vi "Cylinder Chart View.vi"(10 "User Events in":refnum<class "User Events.lvclass">) -> ()   [LabVIEW 2015, in "FAMT Views.lvlib"]
uses:
  FAMT Views.lvlib
  User Events/User Events.lvclass
  User Events/User Events.lvclass/User Events.ctl
  Typedefs/State Types.ctl
  Typedefs/Actuator Types.ctl
  Typedefs/FAMT Typedefs.lvlib
panel:
  out "Chart":T1(graph)
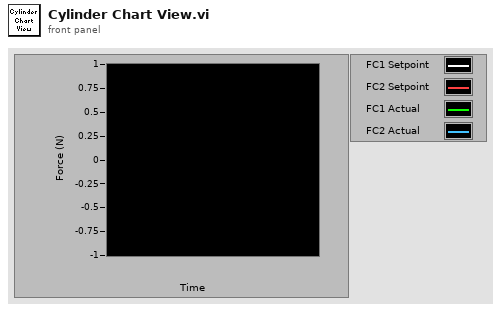
[diagram p1: front panel]
types:
  T1 = cluster{"Axial Demand":dbl, "Lateral Demand":dbl, dbl, dbl}
  T2 = typedef "FAMT Typedefs.lvlib/Publish Data Events.ctl" = cluster{"State":refnum<user-event>, "ErrorCode":refnum<user-event>, "FC1 ILC Outputs":refnum<user-event>, "LogPath":refnum<user-event>, "FC1 ILC Inputs":refnum<user-event>, "Scan Progress":refnum<user-event>, "FC2 ILC Outputs":refnum<user-event>, "FC2 ILC Inputs":refnum<user-event>}
  T3 = cluster{"Event Registration Refnum":refnum<event-registration>, "Event Registration Refnum":refnum<event-registration>}
  T4 = typedef "FAMT Typedefs.lvlib/State Types.ctl" = enum16{"Offline State", "Fault State", "Standby State", "Disabled State", "Enabled State", "Wait For User Input State", "Perform Scan State"}
  T5 = typedef "FAMT Typedefs.lvlib/Actuator Types.ctl" = enum16{"Single", "Dual", "Dual Outer"}
  T6 = cluster{"FC1 Demand":dbl, "FC2 Demand":dbl, dbl, dbl}
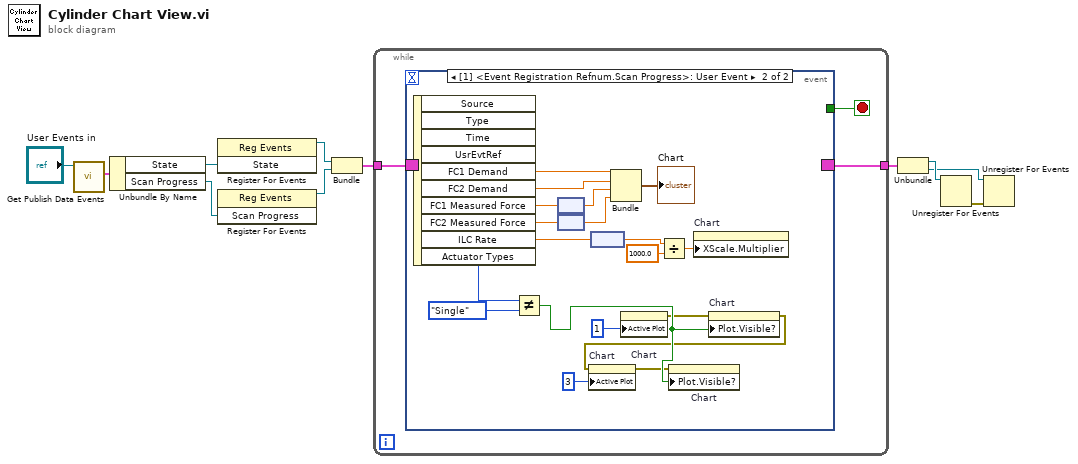
[diagram p0: block diagram]
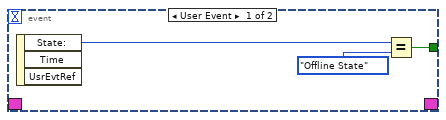
[diagram p2: hidden frame]
diagram:
  n1 = call "Get Publish Data Events.vi"("UserEvents in"="User Events in") -> ("Publish Data Events"=w8:T2)  [unwired: 9 in, 1 out]
  n2 = Unbundle By Name(w8) -> ("State"=w9:refnum<user-event>, "Scan Progress"=w7:refnum<user-event>)
  n3 = register-events(w9) -> (reference out=w11:refnum<event-registration>)  [unwired: 2 in, 1 out]
  n4 = register-events(w7) -> (reference out=w10:refnum<event-registration>)  [unwired: 2 in, 1 out]
  n5 = Bundle("Event Registration Refnum"=w11, "Event Registration Refnum"=w10) -> (w3:T3)  [unwired: 1 in]
  n6 = while {
    tunnel: w3 -> [w14]
    tunnel: [w13] -> w2
    stop <- w12 stop-if-true
    n7 = event shown="[1] <Event Registration Refnum.Scan Progress>: User Event" {
      selector: w14 -> [_ _]
      dyn-events: [_ _] -> w13
      timeout: _ -> [_ _]
      tunnel: [w16 _] -> w12
      event User Event {
        n8 = event-data() -> ("State:"=w15:T4)  [unwired: 1 in, 2 out]
        n9 = Equal?(x=w15, y=State_Types."Offline State") -> (x = y?=w16:bool)
      }
      event User Event {
        n10 = event-data() -> ("FC1 Demand"=w33:dbl, "FC2 Demand"=w27:dbl, "FC1 Measured Force"=w32:dbl[unit], "FC2 Measured Force"=w29:dbl[unit], "ILC Rate"=w26:dbl[unit], "Actuator Types"=w25:T5)  [unwired: 1 in, 4 out]
        n11 = Not Equal?(x=w25, y=Actuator_Types."Single") -> (x != y?=w23:bool)
        n12 = node(w32) -> (w31:dbl)
        n13 = node(w29) -> (w30:dbl)
        n14 = node(w26) -> (w35:dbl)
        n15 = Bundle("FC1 Demand"=w33, "FC2 Demand"=w27, w31, w30) -> (→"Chart":T6)  [unwired: 1 in]
        n16 = property on="Chart" class="WFChart (strict)"("Active Plot"=u32 1) -> (error out=w22:errorcluster)  [unwired: 2 in, 1 out]
        n17 = Divide(x=w35, y=1000.0) -> (x/y=w34:dbl)
        n18 = property on="Chart" class="WFChart (strict)"("XScale.Multiplier"=w34) -> ()  [unwired: 2 in, 2 out]
        n19 = property on="Chart" class="WFChart (strict)"(error in=w22, "Plot.Visible?"=w23) -> (error out=w21:errorcluster)  [unwired: 1 in, 1 out]
        n20 = property on="Chart" class="WFChart (strict)"(error in=w21, "Active Plot"=u32 3) -> (error out=w20:errorcluster)  [unwired: 1 in, 1 out]
        n21 = property on="Chart" class="WFChart (strict)"(error in=w20, "Plot.Visible?"=w23) -> ()  [unwired: 1 in, 2 out]
      }
    }
  }
  n22 = Unbundle(w2) -> ("Event Registration Refnum"=w6:refnum<event-registration>, "Event Registration Refnum"=w5:refnum<event-registration>)
  n23 = Unregister For Events(event registration refnum=w6) -> (error out=w4:errorcluster)  [unwired: 1 in]
  n24 = Unregister For Events(event registration refnum=w5, error in=w4) -> ()  [unwired: 1 out]
